vi "Lower resolution.vi"(10 "Lowest resolution":dbl, 11 "Initial Value":dbl) -> (3 "Coerced value":dbl)   [LabVIEW 2014, in "SLSC configuration System Explorer.lvlib"]
uses:
  SLSC configuration System Explorer.lvlib
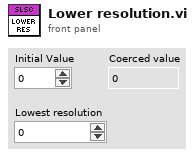
[diagram p1: front panel]
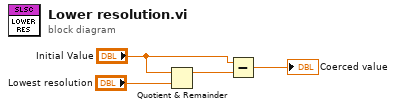
[diagram p0: block diagram]
diagram:
  n1 = Quotient & Remainder(x="Initial Value", y="Lowest resolution") -> (x-y*floor(x/y)=w1:dbl)  [unwired: 1 out]
  n2 = Subtract(x="Initial Value", y=w1) -> (x-y=→"Coerced value":dbl)
